vi "Consolidate Teams and Rankings.vi"(10 "Team List Array":T1, 11 "Team_Scores_And_Rankings_Array":T4(array[cluster])) -> (3 "Consolidated Teams and Rankings":T4(array[cluster]))   [LabVIEW 2013]
uses:
  Round_And_Score_Ctrl.ctl
  Team_List_Array_Ctrl.ctl
  Team_List_Ctrl.ctl
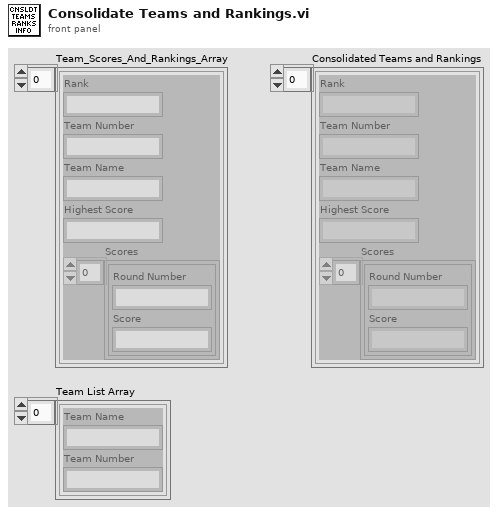
[diagram p1: front panel]
types:
  T1 = typedef "Team_List_Array_Ctrl.ctl" = T2[]
  T2 = typedef "Team_List_Ctrl.ctl" = cluster{"Team Name":string, "Team Number":string}
  T3 = typedef "Round_And_Score_Ctrl.ctl" = cluster{"Score":string, "Round Number":string}
  T4 = cluster{"Rank":string, "Team Number":string, "Team Name":string, "Highest Score":string, "Scores":T3[]}[]
  T5 = cluster{"Rank":string, "Team Number":string, "Team Name":string, "Highest Score":string, "Scores":T3[]}
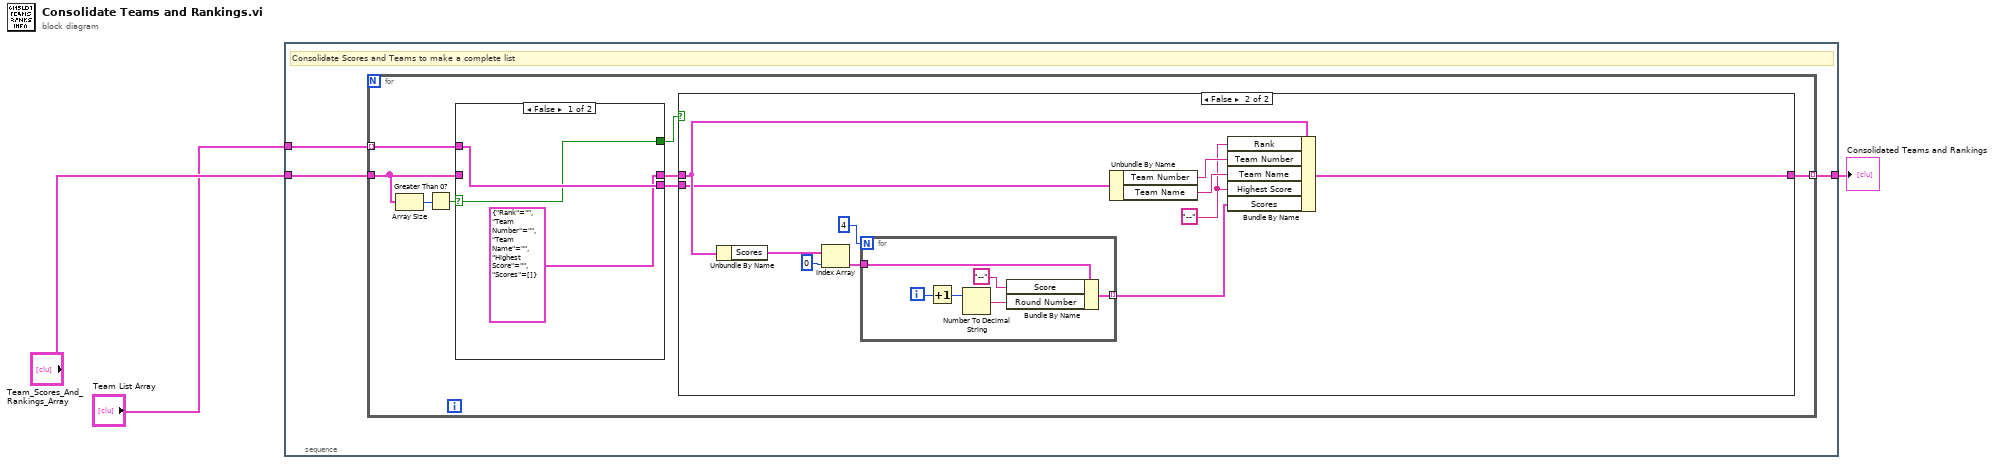
[diagram p0: block diagram]
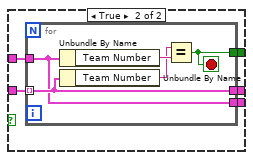
[diagram p2: hidden frame]
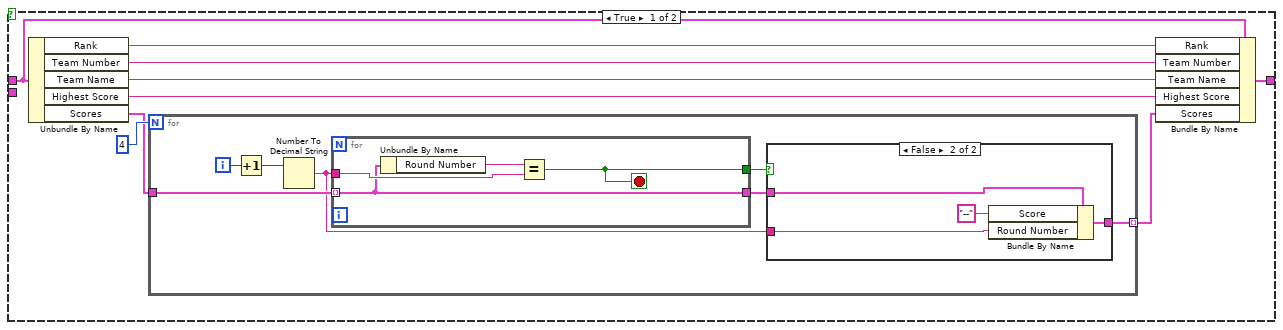
[diagram p3: hidden frame]
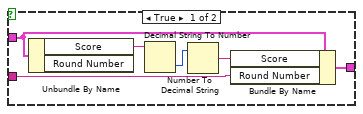
[diagram p4: hidden frame]
diagram:
  n1 = stacked-sequence {
    tunnel: "Team List Array" -> [w6]
    tunnel: "Team_Scores_And_Rankings_Array" -> [w5]
    tunnel: [w4] -> w3
    frame #0 {
      # "Consolidate Scores and Teams to make a complete list"
      n2 = for {
        tunnel: w6 -> [w14] mode=indexing
        tunnel: w5 -> [w7]
        tunnel: [w10] -> w4 mode=indexing
        n3 = Array Size(array=w7) -> (size(s)=w8:i32)
        n4 = Greater Than 0?(x=w8) -> (x > 0?=w9:bool)
        n5 = case shown="False" w9 {
          selector: w9 -> [w15 _]
          tunnel: w14 -> [w17 w22]
          tunnel: w7 -> [_ w21]
          tunnel: [w15 w20] -> w13
          tunnel: [T5 {"Rank"="", "Team Number"="", "Team Name"="", "Highest Score"="", "Scores"=[]} w19] -> w12
          tunnel: [w17 w18] -> w11
          frame False {
          }
          frame True {
            n6 = for {
              tunnel: w22 -> [w23]
              tunnel: w21 -> [w24] mode=indexing
              tunnel: [w25] -> w20
              tunnel: [w24] -> w19
              tunnel: [w23] -> w18
              stop <- w25 stop-if-true
              n7 = Unbundle By Name(w23) -> ("Team Number"=w27:string)
              n8 = Unbundle By Name(w24) -> ("Team Number"=w26:string)
              n9 = Equal?(x=w26, y=w27) -> (x = y?=w25:bool)
            }
          }
        }
        n10 = case shown="False" w13 {
          tunnel: w12 -> [w32 w65]
          tunnel: w11 -> [_ w61]
          tunnel: [w28 w66] -> w10
          frame True {
            n11 = Unbundle By Name(w32) -> ("Rank"=w36:string, "Team Number"=w35:string, "Team Name"=w34:string, "Highest Score"=w33:string, "Scores"=w30:T3[])
            n12 = for {
              N: 4 -> [_]
              tunnel: w30 -> [w42]
              tunnel: [w37] -> w29 mode=indexing
              i -> [w43]
              n13 = Increment(x=w43) -> (x+1=w41:i32)
              n14 = Number To Decimal String(number=w41) -> (decimal integer string=w38:string)  [unwired: 1 in]
              n15 = for {
                tunnel: w42 -> [w54] mode=indexing
                tunnel: w38 -> [w57]
                tunnel: [w55] -> w40
                tunnel: [w54] -> w39
                stop <- w55 stop-if-true
                n16 = Unbundle By Name(w54) -> ("Round Number"=w56:string)
                n17 = Equal?(x=w56, y=w57) -> (x = y?=w55:bool)
              }
              n18 = case shown="False" w40 {
                tunnel: w39 -> [w47 w53]
                tunnel: w38 -> [w45 w52]
                tunnel: [w44 w51] -> w37
                frame True {
                  n19 = Unbundle By Name(w47) -> ("Score"=w49:string)  [unwired: 1 out]
                  n20 = Decimal String To Number(string=w49) -> (number=w48:i32)  [unwired: 2 in, 1 out]
                  n21 = Number To Decimal String(number=w48) -> (decimal integer string=w46:string)  [unwired: 1 in]
                  n22 = Bundle By Name(cluster=w47, "Score"=w46, "Round Number"=w45) -> (w44:T3)
                }
                frame False {
                  n23 = Bundle By Name(cluster=w53, "Score"="--", "Round Number"=w52) -> (w51:T3)
                }
              }
            }
            n24 = Bundle By Name(cluster=w32, "Rank"=w36, "Team Number"=w35, "Team Name"=w34, "Highest Score"=w33, "Scores"=w29) -> (w28:T5)
          }
          frame False {
            w58 = "--" ("Highest Score")
            n25 = Unbundle By Name(w65) -> ("Scores"=w64:T3[])
            n26 = Index Array(array=w64, index=0) -> (element=w63:T3)
            n27 = for {
              N: 4 -> [_]
              tunnel: [w71] -> w67 mode=indexing
              tunnel: w63 -> [w69]
              i -> [w74]
              n28 = Increment(x=w74) -> (x+1=w73:i32)
              n29 = Number To Decimal String(number=w73) -> (decimal integer string=w72:string)  [unwired: 1 in]
              n30 = Bundle By Name(cluster=w69, "Score"="--", "Round Number"=w72) -> (w71:T3)
            }
            n31 = Unbundle By Name(w61) -> ("Team Number"=w60:string, "Team Name"=w59:string)
            n32 = Bundle By Name(cluster=w65, "Rank"=w58, "Team Number"=w60, "Team Name"=w59, "Highest Score"=w58, "Scores"=w67) -> (w66:T5)
          }
        }
      }
    }
  }
  "Consolidated Teams and Rankings" <- w3
